vi "LTVUnicycleCtrl_AtReference.vi"(11 "LTV_UNICYCLE_CONTROLLER":T1={"m_A"=[], "m_B"=[], "m_Q"=[], "m_R"=[], "States"=0, "Inputs"=0, "PoseError"={"TRANSLATION"={"X"=0.0, "Y"=0.0}, "ROTATION"={"VALUE"=0.0, "COS"=1.0, "SIN"=0.0}}, "PoseTolerance"={"TRANSLATION"={"X"=0.0, "Y"=0.0}, "ROTATION"={"VALUE"=0.0, "COS"=1.0, "SIN"=0.0}}, "Dt"=0.02, "Enabled"=FALSE, "savedLQR_K"={"Table Xs"=[], "Table Ys"=[], "MinX"=0.0, "MaxX"=0.0, "ItemCount"=0, "Rows"=0, "Columns"=0}} {"PoseTolerance"."ROTATION"."SIN" format="%13.4f"; "PoseTolerance"."ROTATION"."COS" format="%13.4f"; "PoseTolerance"."ROTATION"."VALUE" format="%13.4f"; "PoseTolerance"."TRANSLATION"."Y" format="%14.3f"; "PoseTolerance"."TRANSLATION"."X" format="%14.3f"; "PoseError"."ROTATION"."SIN" format="%13.4f"; "PoseError"."ROTATION"."COS" format="%13.4f"; "PoseError"."ROTATION"."VALUE" format="%13.4f"; "PoseError"."TRANSLATION"."Y" format="%14.3f"; "PoseError"."TRANSLATION"."X" format="%14.3f"}) -> (3 "At Reference":bool)   [LabVIEW 2019, in "Trajectory_Library.lvlib"]
doc: "Create implicit model follower\n\nInputs:\n - A < states, states > -- Continuous system matrix of the plant being controlled.\n - B < states, inputs > -- Continuous input matrix of the plant being controlled.\n - A_Ref < states, states > -- Continuous system matrix whose dymanics should be followed.\n - B_Ref < states, inputs > -- Continuous input matrix x whose dymanics should be followed.\n\nOutputs:\n - Error -- If TRUE, an error occured."
uses:
  Trajectory_Library.lvlib
  LTV_UNICYCLE_CONTROLLER.ctl
  <vilib>/Analysis/Matrix/Datatypes/RealMatrix.ctl
  POSE2D.ctl
  TRANSLATION2D.ctl
  ROTATION2D.ctl
  FUNCTION_GENERATOR_MATRIX.ctl
  <vilib>/Analysis/Matrix/NI_Matrix.lvlib
panel:
  # "<States,States>"
  # "<States,Inputs>"
  # "<States, States>"
  # "<Inputs, Inputs>"
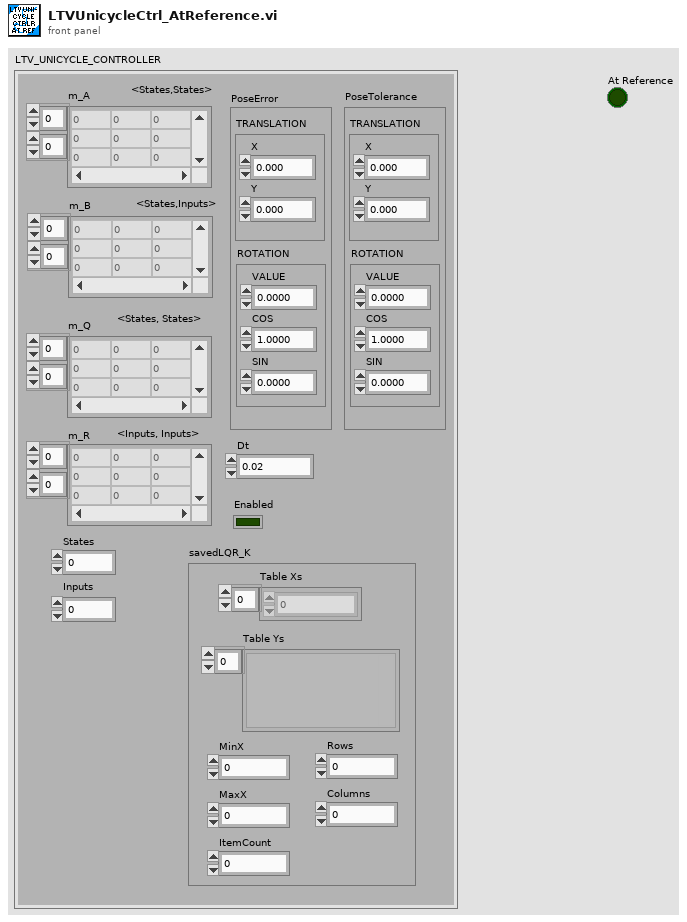
[diagram p1: front panel]
types:
  T1 = typedef "Trajectory_Library.lvlib/LTV_UNICYCLE_CONTROLLER.ctl" = cluster{"m_A":T2, "m_B":T2, "m_Q":T2, "m_R":T2, "States":i32, "Inputs":i32, "PoseError":T3, "PoseTolerance":T3, "Dt":dbl, "Enabled":bool, "savedLQR_K":T6}
  T2 = typedef "NI_Matrix.lvlib/RealMatrix.ctl" = dbl[][]
  T3 = typedef "Trajectory_Library.lvlib/POSE2D.ctl" = cluster{"TRANSLATION":T4, "ROTATION":T5}
  T4 = typedef "Trajectory_Library.lvlib/TRANSLATION2D.ctl" = cluster{"X":dbl, "Y":dbl}
  T5 = typedef "Trajectory_Library.lvlib/ROTATION2D.ctl" = cluster{"VALUE":dbl, "COS":dbl, "SIN":dbl}
  T6 = typedef "Trajectory_Library.lvlib/FUNCTION_GENERATOR_MATRIX.ctl" = cluster{"Table Xs":dbl[], "Table Ys":variant[], "MinX":dbl, "MaxX":dbl, "ItemCount":i32, "Rows":i32, "Columns":i32}
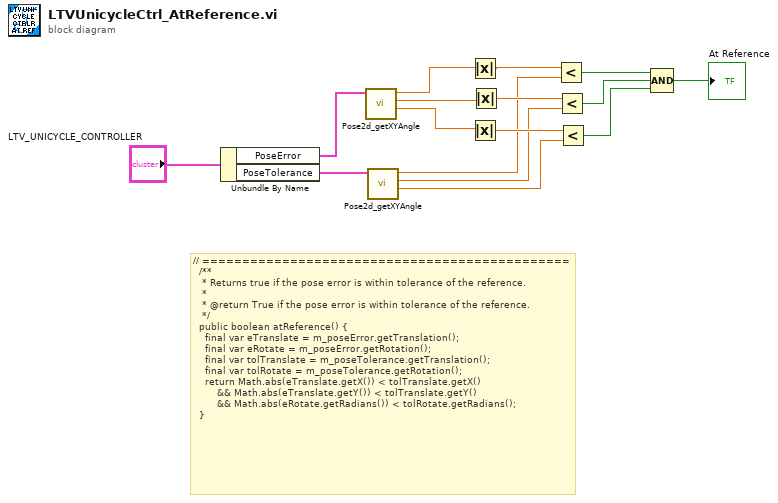
[diagram p0: block diagram]
diagram:
  # "// ==============================================\n  /**\n   * Returns true if the pose error is within tolerance of the reference.\n   *\n   * @return True if the pose error is within tolerance of the reference.\n   */\n  public boolean atReference() {\n    final var eTranslate = m_poseError.getTranslation();\n    final var eRotate = m_poseError.getRotation();\n    final var tolTranslate = m_poseTolerance.getTranslation();\n    final var tolRotate = m_poseTolerance.getRotation();\n    return Math.abs(eTranslate.getX()) < tolTranslate.getX()\n        && Math.abs(eTranslate.getY()) < tolTranslate.getY()\n        && Math.abs(eRotate.getRadians()) < tolRotate.getRadians();\n  }"
  n1 = Unbundle By Name("LTV_UNICYCLE_CONTROLLER") -> ("PoseError"=w15:T3, "PoseTolerance"=w14:T3)
  n2 = call "Pose2d_getXYAngle.vi"("in POSE"=w15) -> ("Angle"=w11:dbl, "Y"=w12:dbl, "X"=w13:dbl)  [unwired: 8 in]
  n3 = call "Pose2d_getXYAngle.vi"("in POSE"=w14) -> ("Angle"=w5:dbl, "Y"=w6:dbl, "X"=w7:dbl)  [unwired: 8 in]
  n4 = Absolute Value(x=w13) -> (abs(x)=w10:dbl)
  n5 = Absolute Value(x=w11) -> (abs(x)=w8:dbl)
  n6 = Absolute Value(x=w12) -> (abs(x)=w9:dbl)
  n7 = Less?(x=w10, y=w7) -> (x < y?=w4:bool)
  n8 = Less?(x=w9, y=w6) -> (x < y?=w3:bool)
  n9 = Less?(x=w8, y=w5) -> (x < y?=w2:bool)
  n10 = Compound Arithmetic op=AND(w4, w3, w2) -> (→"At Reference":bool)
